vi "PostCopyScripting.vi"(10 "MetaDataObj":refnum<class "MetaDataObj.lvclass">, 11 "User Project":refnum<vi>) -> ()   [LabVIEW 2020, in "CCMazeMetaDataObj.lvclass"]
uses:
  CCMazeMetaDataObj.lvclass
  <resource>/dialog/NewProjectWizard/MetaDataObj/MetaDataObj.lvclass
  <vilib>/AppBuilder/AB_API/SDIST/NI_AB_API_SDIST.lvclass
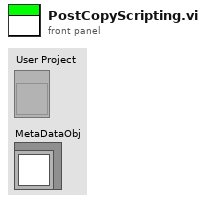
[diagram p1: front panel]
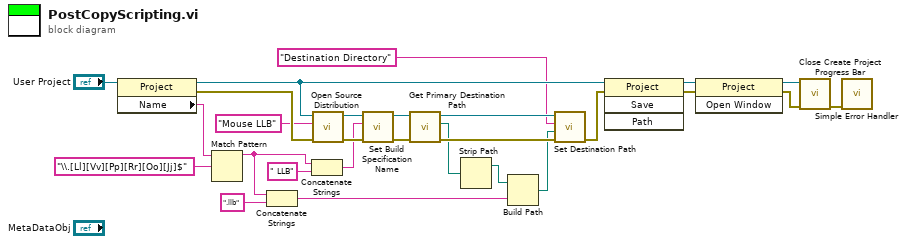
[diagram p0: block diagram]
diagram:
  n1 = property class="Project"(reference="User Project") -> (reference out=w18:refnum<vi>, error out=w25:errorcluster, "Name"=w23:string)  [unwired: 1 in]
  n2 = Match Pattern(string=w23, regular expression="\\.[Ll][Vv][Pp][Rr][Oo][Jj]$") -> (before substring=w15:string)  [unwired: 1 in, 3 out]
  n3 = Concatenate Strings(w15, ".llb" ("string")) -> (w8:string)
  n4 = Concatenate Strings(w15, " LLB" ("string")) -> (w14:string)
  n5 = call <vilib>:"Open Source Distribution.vi"("error in (no error)"=w25, "Build specification name"="Mouse LLB", "Project Refnum"=w18) -> ("error out"=w26:errorcluster, "SDIST out"=w13:refnum<class "NI_AB_API_SDIST.lvclass">)  [unwired: 7 in]
  n6 = call-dynamic "Set Build Specification Name.vi"("error in (no error)"=w26, "Build Specification Name"=w14, "NI_AB_API_SDIST in"=w13) -> ("error out"=w11:errorcluster, "NI_AB_API_SDIST out"=w12:refnum<class "NI_AB_API_SDIST.lvclass">)  [unwired: 7 in]
  n7 = call-dynamic "Get Primary Destination Path.vi"("error in (no error)"=w11, "NI_AB_API_SDIST in"=w12) -> ("error out"=w27:errorcluster, "Primary destination path"=w10:path, "NI_AB_API_SDIST out"=w7:refnum<class "NI_AB_API_SDIST.lvclass">)  [unwired: 7 in]
  n8 = Strip Path(path=w10) -> (stripped path=w9:path)  [unwired: 1 out]
  n9 = Build Path(base path=w9, name or relative path=w8) -> (appended path=w4:path)
  n10 = call-dynamic "Set Destination Path.vi"("error in (no error)"=w27, "Destination path"=w4, "Destination label"="Destination Directory", "SDIST in"=w7) -> ("error out"=w6:errorcluster)  [unwired: 6 in, 1 out]
  n11 = invoke class="Project" method="Save"(reference=w18, error in=w6) -> (reference out=w20:refnum<vi>, error out=w19:errorcluster)  [unwired: 2 in, 2 out]
  n12 = invoke class="Project" method="Open Window"(reference=w20, error in=w19) -> (reference out=w3:refnum<vi>, error out=w2:errorcluster)  [unwired: 1 in, 1 out]
  n13 = call <resource>:"Close Create Project Progress Bar.vi"("error in (no error)"=w2, "Project"=w3) -> ("error out"=w1:errorcluster)  [unwired: 8 in, 1 out]
  n14 = call <vilib>:"Simple Error Handler.vi"("error in (no error)"=w1) -> ()  [unwired: 4 in, 5 out]
